vi "TDC_DAQV_CountingRate_final_rpc.vi"(4 "TDC_ID":u64=3, 6 "Middle ID":u64=1, 7 "bytes to read":i32=1600, 8 "error in (no error)":errorcluster, 9 "UDP Config":bool=TRUE, 10 "timeout":dbl=12.0, 11 "Array":string[](array[string])=["10.3.173.20"]) -> (0 "error out":errorcluster={"status"=TRUE, "code"=56, "source"="TCP Read in TDC_DAQV_CountingRate_final_rpc.vi->电子学自测试.vi"}, 1 "trigger_rate":dbl[](array[numeric])=[-1.0, -1.0, -1.0, -1.0, -1.0, -1.0, -1.0, -1.0, -1.0, -1.0], 2 "time":dbl=8.819787502288818)   [LabVIEW 2017]
panel:
  out "address":string="20"
  out "element":string
  out "substring 4":string
  out "substring 3":string
  out "Histogram":dynamicdata(graph)=[{"t0"=timestamp(0.5 s since 1904-01-01), "dt"=1.0, "Y"=[291.0, 0.0, 0.0, 0.0, 1.0, 0.0, 0.0, 0.0, 1.0, 0.0, 0.0, 0.0, 0.0, 0.0, 0.0, 0.0, 0.0, 0.0, 0.0, 0.0, 0.0, 0.0, 0.0, 0.0, 1.0, 0.0, 0.0, 0.0, 3.0, 0.0, 0.0, 0.0, 3.0, 0.0, 0.0, 0.0, 0.0, 0.0, 0.0, 0.0, 0.0, 0.0, 0.0, 0.0, 0.0, 0.0, 0.0, 0.0, 0.0, 0.0, 0.0, 0.0, 0.0, 0.0, 0.0, 0.0, 0.0, 0.0, 0.0, 0.0, 0.0, 0.0, 0.0, 0.0, 0.0, 0.0, 0.0, 0.0, 0.0, 0.0, 0.0, 0.0, 0.0, 0.0, 0.0, 0.0, 0.0, 0.0, 0.0, 0.0], "attributes"=variant("NI_ChannelName"=variant(string " (Histogram)"), "NI_ExpIsRelativeTime"=variant(bool TRUE), "NI_ExpStartTimeStamp"=variant(timestamp timestamp(0 s since 1904-01-01)), "NI_ExpTimeStamp"=variant(timestamp timestamp(0 s since 1904-01-01)), "NI_ExpXDimension"=variant(string "BIN"), "NI_OriginalChannelName"=variant(string ""))}] caption="直方图"
  out "求和":dbl=-10.0
  out "PAD NO":u64
  in  "Thresholds":dbl=-0.03
  in  "one key for threshold":bool=TRUE
  in  "SMA mode":bool
  in  "Thresholds (mV)":dbl[](array[numeric])=[580.0, 580.0, 580.0, 580.0, 600.0, 600.0, 600.0, 600.0, 580.0, 580.0, 600.0, 600.0, 600.0, 600.0, 600.0, 600.0, 580.0, 580.0, 600.0, 600.0, 600.0, 600.0, 600.0, 600.0, 580.0, 580.0, 600.0, 600.0, 600.0, 600.0, 600.0, 600.0, 600.0, 600.0, 600.0, 600.0, 600.0, 600.0, 600.0, 600.0, 600.0, 600.0, 600.0, 600.0, 600.0, 600.0, 600.0, 600.0, 600.0, 600.0, 600.0, 600.0, 600.0, 600.0, 600.0, 600.0, 600.0, 600.0, 600.0, 600.0, 600.0, 600.0, 600.0, 600.0]
  out "Out":u8=3 format="%.0x"
  out "substring 2":string
  out "array":dbl[](array[numeric])=[-1.0, -1.0, -1.0, -1.0, -1.0, -1.0, -1.0, -1.0, -1.0, -1.0]
  out "trigger number":u64 format="%x"
  out "number":u32
  in  "factor":i32=2
  in  "stop":bool
  in  "timeout (ms)":i32=8400
  # "5A00 0000 0000 03E8 FC38 000B 800F 3F7B"
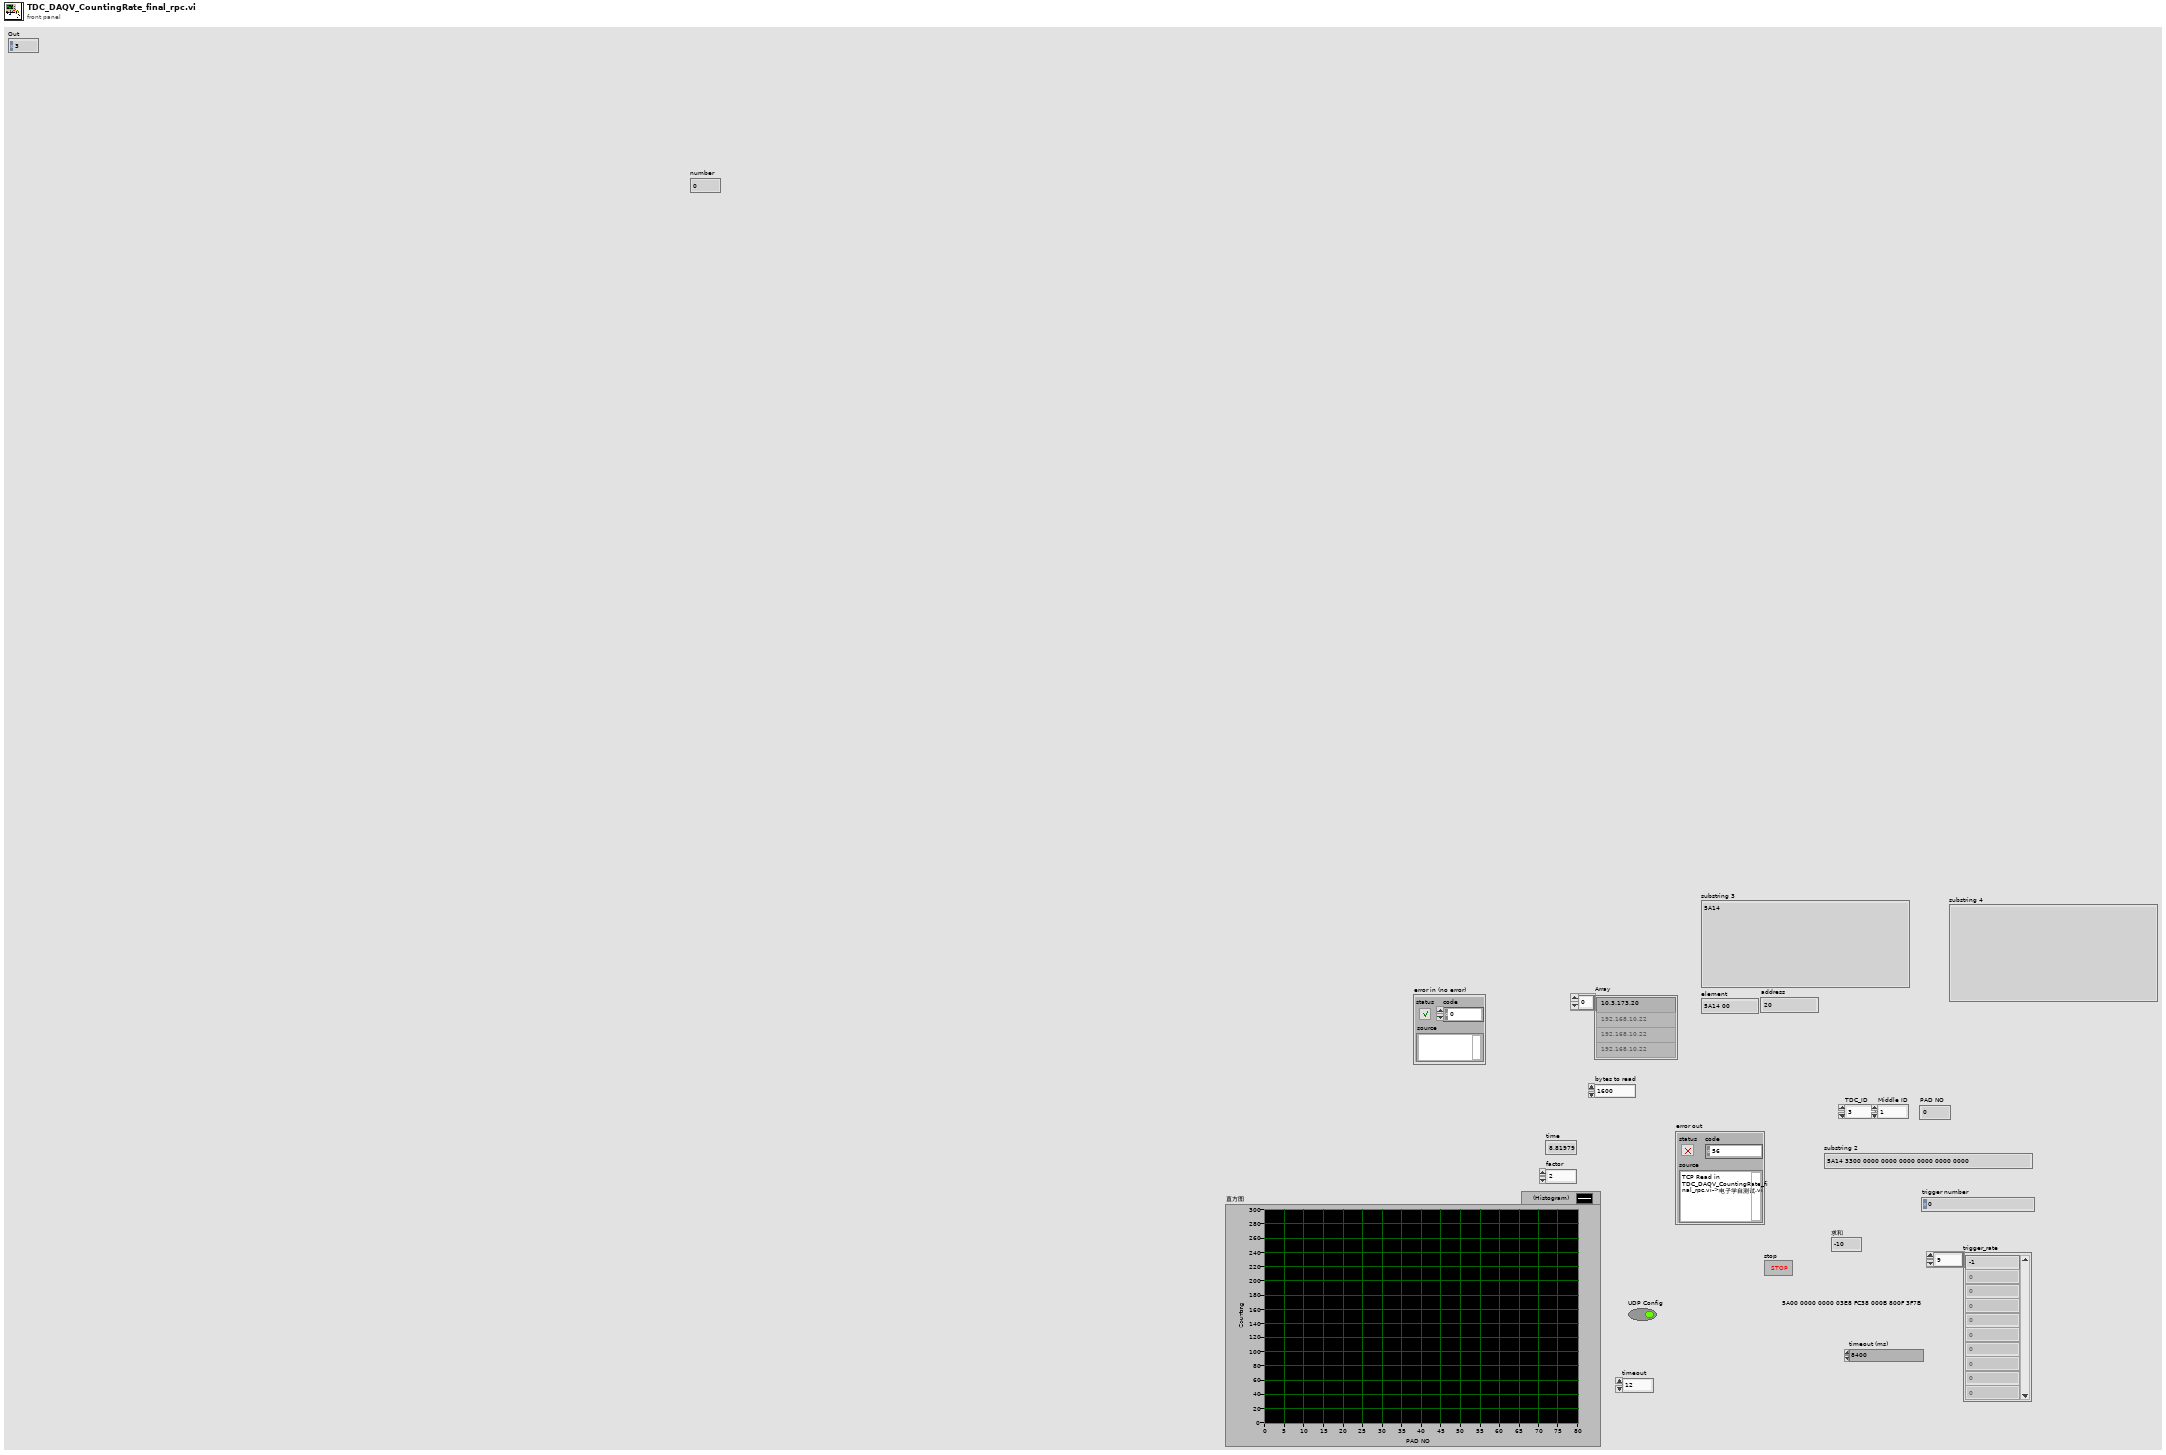
[diagram p1: front panel]
types:
  T1 = enum16{"Standard", "Buffered", "CRLF", "Immediate"}
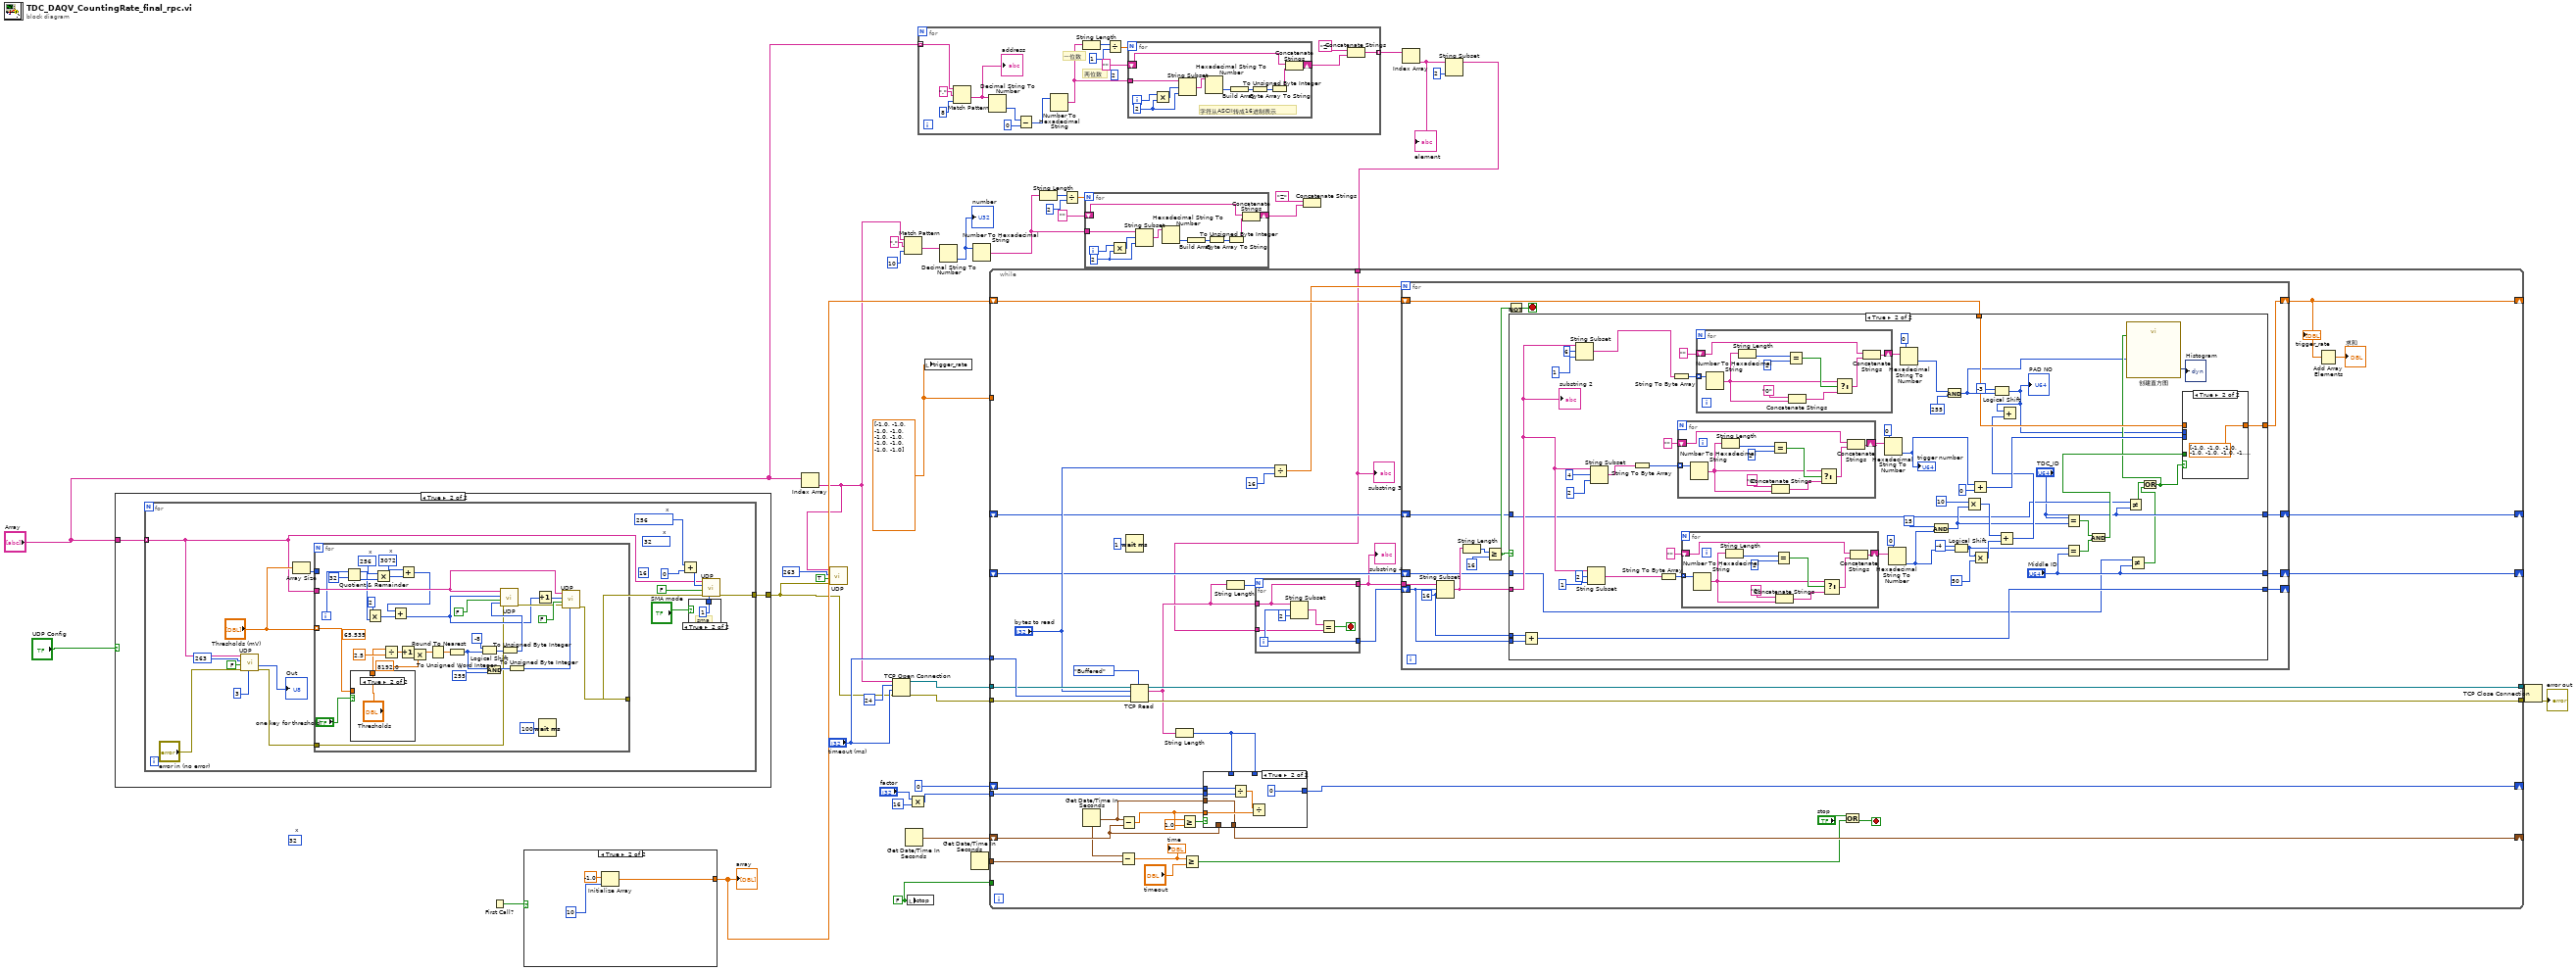
[diagram p0: block diagram]
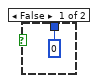
[diagram p3: hidden frame]
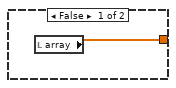
[diagram p5: hidden frame]
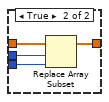
[diagram p8: hidden frame]
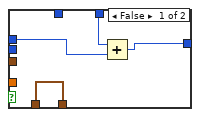
[diagram p9: hidden frame]
diagram:
  w11 = dbl[] [-1.0, -1.0, -1.0, -1.0, -1.0, -1.0, -1.0, -1.0, -1.0, -1.0] ("rate_array")
  w26 = FALSE ("stop")
  (unwired) u16 32  # x
  n1 = case shown="True" "UDP Config" {
    tunnel: "Array" -> [_ w39]
    tunnel: [_ w40] -> w4
    frame False {
    }
    frame True {
      n2 = for {
        tunnel: [w55] -> w40
        tunnel: w39 -> [w43] mode=indexing
        (unwired) u16 32  # x
        (unwired) u32 16 ("Address")
        w48 = u16 256  # x
        n3 = call "UDP.vi"("In"=u8 3, "error in (no error)"="error in (no error)", "Read (TRUE)"=FALSE, "Address"=u32 263, "IP address"=w43) -> ("error out"=w41:errorcluster, "Out"=→"Out":u8)  [unwired: 3 in, 1 out]
        n4 = Array Size(array="Thresholds (mV)") -> (size(s)=w52:i32)
        n5 = for {
          tunnel: w43 -> [w89]
          tunnel: "Thresholds (mV)" -> [w76] mode=indexing
          tunnel: [w79] -> w56
          tunnel: w52 -> [_]
          tunnel: w41 -> [w63]
          i -> [w71]
          (unwired) 65.535 ("y")
          w72 = u16 3072  # x
          w73 = u16 256  # x
          w85 = u16 255  # x
          n6 = Quotient & Remainder(x=w71, y=32) -> (x-y*floor(x/y)=w65:i32, floor(x/y)=w74:i32)
          n7 = case shown="True" "one key for threshold" {
            tunnel: [w95 "Thresholds"] -> w77
            tunnel: w76 -> [w95 _]
            frame False {
            }
            frame True {
            }
          }
          n8 = Multiply(x=2, y=w65) -> (x*y=w66:i32)
          n9 = Multiply(x=w73, y=w74) -> (x*y=w68:i32)
          n10 = Divide(x=w77, y=2.5) -> (x/y=w92:dbl)
          n11 = Increment(x=w92) -> (x+1=w62:dbl)
          n12 = Add(x=w72, y=w68) -> (x+y=w67:i32)
          n13 = Add(x=w67, y=w66) -> (x+y=w70:i32)
          n14 = Multiply(x=w62, y=8192.0) -> (x*y=w61:dbl)
          n15 = Round To Nearest(number=w61) -> (nearest integer value=w90:dbl)
          n16 = To Unsigned Word Integer(number=w90) -> (unsigned 16bit integer=w81:u16)
          n17 = Logical Shift(y=i16 -8, x=w81) -> (x << y=w87:u16)
          n18 = And(x=w81, y=w85) -> (x .and. y?=w84:u16)
          n19 = To Unsigned Byte Integer(number=w87) -> (unsigned 8bit integer=w86:u8)
          n20 = call "UDP.vi"("In"=w86, "error in (no error)"=w63, "Read (TRUE)"=FALSE, "Address"=w70, "IP address"=w89) -> ("error out"=w80:errorcluster)  [unwired: 3 in, 2 out]
          n21 = To Unsigned Byte Integer(number=w84) -> (unsigned 8bit integer=w83:u8)
          n22 = Increment(x=w70) -> (x+1=w69:i32)
          n23 = Wait (ms)(milliseconds to wait=u32 100) -> ()  [unwired: 1 out]
          n24 = call "UDP.vi"("In"=w83, "error in (no error)"=w80, "Read (TRUE)"=FALSE, "Address"=w69, "IP address"=w89) -> ("error out"=w79:errorcluster)  [unwired: 3 in, 2 out]
        }
        n25 = Add(x=w48, y=u32 0 ("Address")) -> (x+y=w49:u32)
        n26 = case shown="True" "SMA mode" {
          tunnel: [u8 0 ("In") u8 1 ("In")] -> w54
          frame False {
          }
          frame True {
            # "sma"
          }
        }
        n27 = call "UDP.vi"("In"=w54, "error in (no error)"=w56, "Read (TRUE)"=FALSE, "Address"=w49, "IP address"=w43) -> ("error out"=w55:errorcluster)  [unwired: 3 in, 2 out]
      }
    }
  }
  n28 = First Call?() -> (First Call?: T/F=w13:bool)
  n29 = case shown="True" w13 {
    tunnel: [w97 w98] -> w12
    frame False {
      n30 = local read "array"() -> (w97:dbl[])
    }
    frame True {
      n31 = Initialize Array(-1.0 ("element"), 10 ("dimension size")) -> (w98:dbl[])
    }
  }
  "array" <- w12
  n32 = Index Array(array="Array") -> (element=w3:string)  [unwired: 1 in]
  n33 = call "UDP.vi"("error in (no error)"=w4, "Read (TRUE)"=TRUE, "Address"=u32 263, "IP address"=w3) -> ()  [unwired: 4 in, 3 out]
  n34 = TCP Open Connection(address=w3, remote port or service name=u16 24 ("port"), timeout ms (60000)="timeout (ms)", error in (no error)=w4) -> (connection ID=w36:refnum<k5>, error out=w37:errorcluster)  [unwired: 1 in]
  n35 = Match Pattern(string=w3, regular expression="." ("search string"), offset (0)=10) -> (after substring=w17:string)  [unwired: 3 out]
  n36 = Get Date/Time In Seconds() -> (seconds since 1Jan1904=w32:timestamp)
  n37 = local write "stop"(w26) -> ()
  n38 = Multiply(x="factor", y=16) -> (x*y=w28:i32)
  n39 = for {
    tunnel: [w103] -> w8 mode=indexing
    tunnel: "Array" -> [w102] mode=indexing
    (unwired) 2 ("y")
    # "一位数"
    # "两位数"
    n40 = Match Pattern(string=w102, regular expression="." ("search string"), offset (0)=8) -> (after substring=w101:string)  [unwired: 3 out]
    "address" <- w101
    n41 = Decimal String To Number(string=w101) -> (number=w106:i32)  [unwired: 2 in, 1 out]
    n42 = Subtract(x=w106, y=0) -> (x-y=w105:i32)
    n43 = Number To Hexadecimal String(2:w105) -> (0:w108:string)  [unwired: 1 in]
    n44 = String Length(string=w108) -> (length=w113:i32)
    n45 = Divide(x=w113, y=1) -> (x/y=w114:dbl)
    n46 = for {
      N: w114 -> [_]
      shift-right: [w126] -> w104
      shift-left: "" ("format string") -> [w125]
      tunnel: w108 -> [w116]
      i -> [w124]
      w118 = 2 ("y")
      # "字符从ASCII转成16进制表示"
      n47 = Multiply(x=w124, y=w118) -> (x*y=w117:i32)
      n48 = String Subset(string=w116, offset (0)=w117, length (rest)=w118) -> (substring=w119:string)
      n49 = Hexadecimal String To Number(string=w119) -> (number=w123:u32)  [unwired: 2 in, 1 out]
      n50 = Build Array(w123) -> (w122:u32[])
      n51 = To Unsigned Byte Integer(number=w122) -> (unsigned 8bit integer=w121:u8[])
      n52 = Byte Array To String(unsigned byte array=w121) -> (string=w120:string)
      n53 = Concatenate Strings(w125, w120) -> (w126:string)
    }
    n54 = Concatenate Strings("Z", w104) -> (w103:string)
  }
  n55 = local write "trigger_rate"(w11) -> ()
  n56 = Decimal String To Number(string=w17) -> (number=w16:i32)  [unwired: 2 in, 1 out]
  "number" <- w16
  n57 = Get Date/Time In Seconds() -> (seconds since 1Jan1904=w25:timestamp)
  n58 = Number To Hexadecimal String(2:w16) -> (0:w15:string)  [unwired: 1 in]
  n59 = String Length(string=w15) -> (length=w22:i32)
  n60 = Divide(x=w22, y=2) -> (x/y=w23:dbl)
  n61 = for {
    N: w23 -> [_]
    shift-right: [w137] -> w14
    shift-left: "" ("format string") -> [w136]
    tunnel: w15 -> [w127]
    i -> [w135]
    w129 = 2 ("y")
    n62 = Multiply(x=w135, y=w129) -> (x*y=w128:i32)
    n63 = String Subset(string=w127, offset (0)=w128, length (rest)=w129) -> (substring=w130:string)
    n64 = Hexadecimal String To Number(string=w130) -> (number=w134:u32)  [unwired: 2 in, 1 out]
    n65 = Build Array(w134) -> (w133:u32[])
    n66 = To Unsigned Byte Integer(number=w133) -> (unsigned 8bit integer=w132:u8[])
    n67 = Byte Array To String(unsigned byte array=w132) -> (string=w131:string)
    n68 = Concatenate Strings(w136, w131) -> (w137:string)
  }
  n69 = Concatenate Strings("Z", w14) -> ()  [unwired: 1 out]
  n70 = Index Array(array=w8) -> (element=w7:string)  [unwired: 1 in]
  "element" <- w7
  n71 = String Subset(string=w7, length (rest)=2 ("长度（剩余）")) -> (substring=w2:string)  [unwired: 1 in]
  n72 = while {
    tunnel: w37 -> [w175]
    tunnel: "timeout (ms)" -> [w174]
    tunnel: w36 -> [w173]
    tunnel: [w172] -> w35
    tunnel: [w171] -> w34
    shift-right: [w164] -> _
    shift-left: w32 -> [w168]
    shift-right: [w167] -> _
    shift-left: u32 0 ("milliseconds to wait") -> [w162]
    tunnel: w28 -> [w161]
    tunnel: w26 -> [_]
    tunnel: w25 -> [w155]
    tunnel: w2 -> [w138]
    shift-right: [w145] -> _
    shift-left: w12 -> [w150]
    tunnel: w11 -> [_]
    shift-right: [w142] -> _
    shift-left: _ -> [w140]
    shift-right: [w143] -> _
    shift-left: _ -> [w141]
    stop <- w158 stop-if-true
    n73 = Get Date/Time In Seconds() -> (seconds since 1Jan1904=w154:timestamp)
    n74 = Subtract(x=w154, y=w155) -> (x-y=w153:dbl)
    "time" <- w153
    n75 = Subtract(x=w154, y=w168) -> (x-y=w160:dbl)
    n76 = Wait (ms)(milliseconds to wait=u32 1) -> ()  [unwired: 1 out]
    n77 = TCP Read(connection ID=w173, bytes to read="bytes to read", error in (no error)=w175, 7:T1."Buffered" ("mode (standard)"), 9:w174) -> (connection ID out=w172:refnum<k5>, data out=w151:string, error out=w171:errorcluster)
    n78 = String Length(string=w151) -> (length=w163:i32)
    n79 = Greater Or Equal?(x=w160, y=1.0) -> (x >= y?=w166:bool)
    n80 = Greater Or Equal?(x=w153, y="timeout") -> (x >= y?=w156:bool)
    n81 = case shown="True" w166 {
      tunnel: w160 -> [_ w307]
      tunnel: w154 -> [_ w306]
      tunnel: [w301 w306] -> w164
      tunnel: w168 -> [w301 _]
      tunnel: w163 -> [_ _]
      tunnel: w163 -> [w300 _]
      tunnel: [w299 0] -> w167
      tunnel: w161 -> [_ w303]
      tunnel: w162 -> [w298 w302]
      frame False {
        n82 = Add(x=w300, y=w298) -> (x+y=w299:u32)
      }
      frame True {
        n83 = Divide(x=w302, y=w303) -> (x/y=w305:dbl)
        n84 = Divide(x=w305, y=w307) -> ()  [unwired: 1 out]
      }
    }
    n85 = String Length(string=w151) -> (length=w152:i32)
    n86 = for {
      N: w152 -> [_]
      tunnel: w151 -> [w294]
      tunnel: [w294] -> w139
      tunnel: [w293] -> w149
      tunnel: w138 -> [w292]
      i -> [w293]
      stop <- w295 stop-if-true
      n87 = String Subset(string=w294, offset (0)=w293, length (rest)=2 ("length (rest)")) -> (substring=w296:string)
      n88 = Equal?(x=w296, y=w292) -> (x = y?=w295:bool)
    }
    "substring 4" <- w139
    n89 = Divide(x="bytes to read", y=16 ("length (rest)")) -> (x/y=w146:dbl)
    n90 = for {
      N: w146 -> [_]
      tunnel: w139 -> [w190]
      shift-right: [w188] -> w145
      shift-left: w150 -> [w189]
      shift-right: [w180] -> _
      shift-left: w149 -> [w181]
      shift-right: [w179] -> w143
      shift-left: w141 -> [w176]
      shift-right: [w178] -> w142
      shift-left: w140 -> [w177]
      stop <- w183 stop-if-true
      w182 = 16 ("length (rest)")
      n91 = String Subset(string=w190, offset (0)=w181, length (rest)=w182) -> (substring=w187:string)
      n92 = String Length(string=w187) -> (length=w186:i32)
      n93 = Greater Or Equal?(x=w186, y=16 ("length (rest)")) -> (x >= y?=w184:bool)
      n94 = Not(x=w184) -> (.not. x?=w183:bool)
      n95 = case shown="True" w184 {
        tunnel: w187 -> [_ w232]
        tunnel: w189 -> [w194 w231]
        tunnel: [w194 w230] -> w188
        tunnel: w181 -> [w193 w229]
        tunnel: w182 -> [_ w228]
        tunnel: [w193 w227] -> w180
        tunnel: [w192 "TDC_ID"] -> w179
        tunnel: [w191 "Middle ID"] -> w178
        tunnel: w177 -> [w191 w200]
        tunnel: w176 -> [w192 w204]
        frame False {
        }
        frame True {
          n96 = Add(x=w228, y=w229) -> (x+y=w227:i32)
          n97 = String Subset(string=w232, offset (0)=6, length (rest)=1 ("length (rest)")) -> (substring=w235:string)
          n98 = String Subset(string=w232, offset (0)=2, length (rest)=1 ("length (rest)")) -> (substring=w222:string)
          n99 = String Subset(string=w232, offset (0)=4, length (rest)=2 ("length (rest)")) -> (substring=w242:string)
          n100 = String To Byte Array(string=w242) -> (unsigned byte array=w244:u8[])
          n101 = String To Byte Array(string=w222) -> (unsigned byte array=w225:u8[])
          n102 = String To Byte Array(string=w235) -> (unsigned byte array=w238:u8[])
          n103 = for {
            shift-right: [w290] -> w245
            shift-left: "" ("format string") -> [w287]
            tunnel: w244 -> [w291] mode=indexing
            n104 = Number To Hexadecimal String(2:w291) -> (0:w283:string)  [unwired: 1 in]
            n105 = String Length(string=w283) -> (length=w289:i32)
            n106 = Equal?(x=w289, y=2) -> (x = y?=w286:bool)
            n107 = Concatenate Strings("0" ("format string"), w283) -> (w285:string)
            n108 = Select(t=w283, s=w286, f=w285) -> (s? t:f=w282:string)
            n109 = Concatenate Strings(w287, w282) -> (w290:string)
          }
          n110 = for {
            shift-right: [w270] -> w224
            shift-left: "" ("format string") -> [w267]
            tunnel: w225 -> [w271] mode=indexing
            n111 = Number To Hexadecimal String(2:w271) -> (0:w263:string)  [unwired: 1 in]
            n112 = String Length(string=w263) -> (length=w269:i32)
            n113 = Equal?(x=w269, y=2) -> (x = y?=w266:bool)
            n114 = Concatenate Strings("0" ("format string"), w263) -> (w265:string)
            n115 = Select(t=w263, s=w266, f=w265) -> (s? t:f=w262:string)
            n116 = Concatenate Strings(w267, w262) -> (w270:string)
          }
          n117 = for {
            shift-right: [w280] -> w237
            shift-left: "" ("format string") -> [w277]
            tunnel: w238 -> [w281] mode=indexing
            n118 = Number To Hexadecimal String(2:w281) -> (0:w273:string)  [unwired: 1 in]
            n119 = String Length(string=w273) -> (length=w279:i32)
            n120 = Equal?(x=w279, y=2) -> (x = y?=w276:bool)
            n121 = Concatenate Strings("0" ("format string"), w273) -> (w275:string)
            n122 = Select(t=w273, s=w276, f=w275) -> (s? t:f=w272:string)
            n123 = Concatenate Strings(w277, w272) -> (w280:string)
          }
          n124 = Hexadecimal String To Number(string=w245, default (0uL)=u64 0 ("default (0 U32)")) -> (number=w220:u64)  [unwired: 1 in, 1 out]
          "trigger number" <- w220
          n125 = Hexadecimal String To Number(string=w224, default (0uL)=u64 0 ("default (0 U32)")) -> (number=w215:u64)  [unwired: 1 in, 1 out]
          n126 = Hexadecimal String To Number(string=w237, default (0uL)=u64 0 ("default (0 U32)")) -> (number=w234:u64)  [unwired: 1 in, 1 out]
          n127 = And(x=u64 15 ("default (0 U32)"), y=w215) -> (x .and. y?=w209:u64)
          n128 = And(x=w234, y=u64 255 ("default (0 U32)")) -> (x .and. y?=w196:u64)
          n129 = Logical Shift(y=i16 -4, x=w215) -> (x << y=w208:u64)
          n130 = Multiply(x=u64 10, y=w209) -> (x*y=w211:u64)
          n131 = Add(x=w220, y=u64 0) -> (x+y=w219:u64)
          n132 = Multiply(x=w208, y=u64 50 ("x")) -> (x*y=w212:u64)
          n133 = Logical Shift(y=i16 -3, x=w196) -> (x << y=w195:u64)
          "PAD NO" <- w195
          n134 = Add(x=w211, y=w212) -> (x+y=w210:u64)
          n135 = Add(x=w195, y=w210) -> ()  [unwired: 1 out]
          n136 = Equal?(x="TDC_ID", y=w209) -> (x = y?=w206:bool)
          n137 = Equal?(x=w208, y="Middle ID") -> (x = y?=w207:bool)
          n138 = And(x=w206, y=w207) -> (x .and. y?=w205:bool)
          n139 = Not Equal?(x=w204, y="TDC_ID") -> (x != y?=w202:bool)
          n140 = Not Equal?(x=w200, y="Middle ID") -> (x != y?=w199:bool)
          n141 = Or(x=w202, y=w199) -> (x .or. y?=w198:bool)
          n142 = call "创建直方图"("Reset"=w198, "Signal"=w196) -> ("Histogram"=→"Histogram":dynamicdata)  [unwired: 8 in, 1 out]
          n143 = case shown="True" w198 {
            tunnel: w231 -> [w255 _]
            tunnel: [w254 dbl[] [-1.0, -1.0, -1.0, -1.0, -1.0, -1.0, -1.0, -1.0, -1.0, -1.0] ("rate_array")] -> w230
            tunnel: w219 -> [w253 _]
            tunnel: w195 -> [w252 _]
            tunnel: w205 -> [w251 _]
            frame False {
              n144 = case shown="False" w251 {
                tunnel: w255 -> [w256 w260]
                tunnel: [w256 w259] -> w254
                tunnel: w253 -> [_ w258]
                tunnel: w252 -> [_ w257]
                frame False {
                }
                frame True {
                  n145 = Replace Array Subset(array=w260, new element=w258, index=w257) -> (w259:dbl[])
                }
              }
            }
            frame True {
            }
          }
          "substring 2" <- w232
        }
      }
    }
    "trigger_rate" <- w145
    n146 = Or(x="stop", y=w156) -> (x .or. y?=w158:bool)
    n147 = Add Array Elements(numeric array=w145) -> (sum=→"求和":dbl)
    "substring 3" <- w138
  }
  n148 = TCP Close Connection(connection ID=w35, error in (no error)=w34) -> (error out=→"error out":errorcluster)  [unwired: 1 in, 1 out]
